vi "PlantZ.vi"(4 "uk":dbl format="%#_13g") -> (1 "yk":dbl)   [LabVIEW 2015]
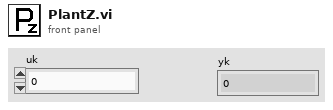
[diagram p1: front panel]
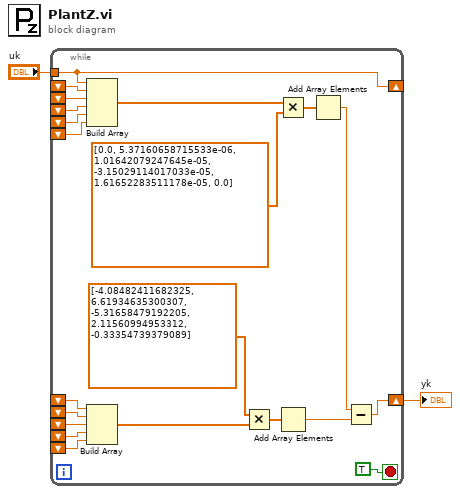
[diagram p0: block diagram]
diagram:
  n1 = while {
    tunnel: "uk" -> [w14]
    shift-right: [w14] -> _
    shift-left: _ -> [w13]
    shift-left: _ -> [w12]
    shift-left: _ -> [w11]
    shift-left: _ -> [w10]
    shift-left: _ -> [w9]
    shift-right: [w8] -> w1
    shift-left: _ -> [w7]
    shift-left: _ -> [w6]
    shift-left: _ -> [w5]
    shift-left: _ -> [w4]
    shift-left: _ -> [w3]
    stop <- TRUE stop-if-true
    n2 = Build Array(w14, w13, w12, w11, w10, w9) -> (w17:dbl[])
    n3 = Build Array(w7, w6, w5, w4, w3) -> (w22:dbl[])
    n4 = Multiply(x=dbl[] [-4.08482411682325, 6.61934635300307, -5.31658479192205, 2.11560994953312, -0.33354739379089] ("Qd"), y=w22) -> (x*y=w20:dbl[])
    n5 = Multiply(x=w17, y=dbl[] [0.0, 5.37160658715533e-06, 1.01642079247645e-05, -3.15029114017033e-05, 1.61652283511178e-05, 0.0] ("Qd")) -> (x*y=w18:dbl[])
    n6 = Add Array Elements(numeric array=w20) -> (sum=w21:dbl)
    n7 = Add Array Elements(numeric array=w18) -> (sum=w19:dbl)
    n8 = Subtract(x=w19, y=w21) -> (x-y=w8:dbl)
  }
  "yk" <- w1
